vi "4-channel arduino.vi"() -> ()   [LabVIEW 2014]
uses:
  <vilib>/MakerHub/LINX/Public/Peripherals/Analog/Analog Read 1 Chan.vi
  <vilib>/MakerHub/LINX/LMH-LINX.lvlib
panel:
  out "Numeric":dbl
  in  "AI Channel 4":u8
  in  "AI Channel 3":u8
  in  "AI Channel 2":u8
  in  "AI Channel 1":u8
  in  "AI Channel 0":u8
  in  "Stop Button":bool
  out "Analog Data 0":dbl(graph)
  out "Loop Rate (Hz)":u32
  out "Analog Data 1":dbl(graph)
  out "Analog Data 2":dbl(graph)
  out "Analog Data 3":dbl(graph)
  out "Analog Data 4":dbl(graph)
  in  "Serial Port":refnum<visa-resource-name>
  # "Analog Data 0"
  # "Analog Data 1"
  # "Analog Data 4"
  # "Analog Data 2"
  # "Analog Data 3"
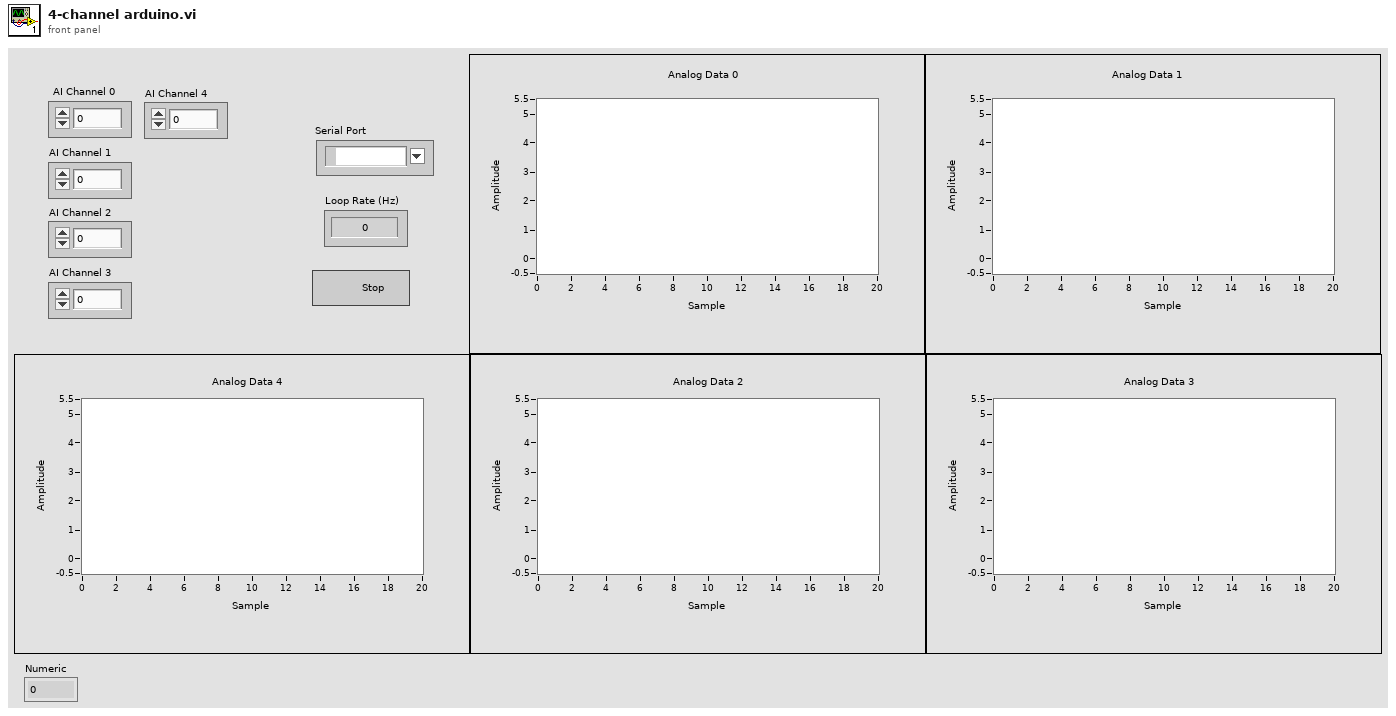
[diagram p1: front panel]
types:
  T1 = typedef "LMH-LINX.lvlib/LINX Ref.ctl" = cluster{"Platform":T2, "Interface":T3, "LINX Device Config":T4}
  T2 = typedef "LMH-LINX.lvlib/Platform.ctl" = enum16{"LINX", "myRIO"}
  T3 = typedef "LMH-LINX.lvlib/Interface.ctl" = enum16{"Serial", "TCP"}
  T4 = typedef "LMH-LINX.lvlib/Device.lvlib/LINX Device Config.ctl" = cluster{"Interface":T3, "COM Port":refnum<visa-resource-name>, "TCP Configuration":T5, "Device Family":u8, "Device ID":u8, "Device Name":string, "TCP Ref":refnum<k5>, "Channels":T6}
  T5 = typedef "LMH-LINX.lvlib/Device.lvlib/TCP Config.ctl" = cluster{"IP Address":string, "Port":u16}
  T6 = typedef "LMH-LINX.lvlib/Channels.ctl" = cluster{"DI":u8[], "DO":u8[], "AI":u8[], "AO":u8[], "PWM":u8[], "QE":u8[], "UART":u8[], "I2C 2":u8[], "SPI":u8[], "CAN":u8[], "Servo":u8[], "AI Ref (V)":dbl, "AO Ref (V)":dbl, "AO Resolution (Bits)":u8}
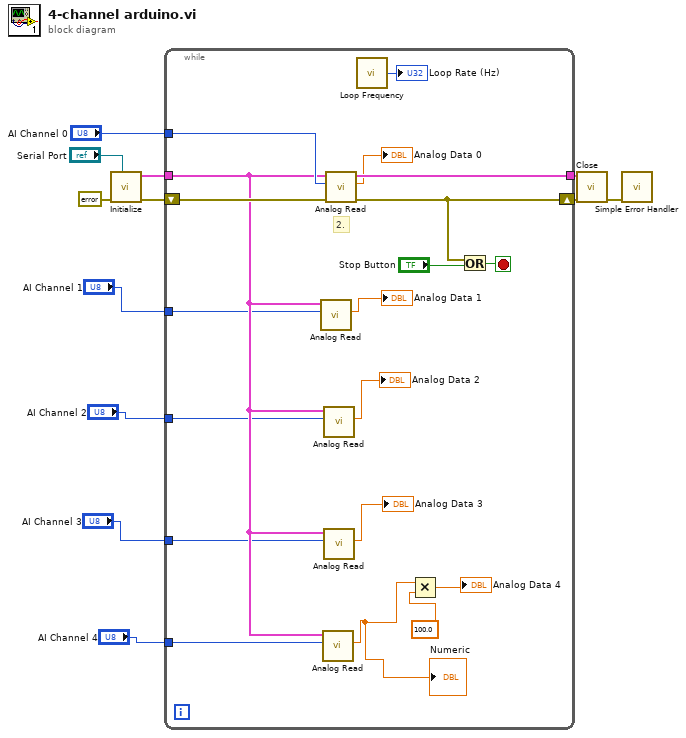
[diagram p0: block diagram]
diagram:
  n1 = call <vilib>:"Initialize.vi"("Serial Port"="Serial Port", "Error In"=errorcluster {"status"=FALSE, "code"=0, "source"=""}) -> ("Error Out"=w11:errorcluster, "LINX Ref"=w12:T1)  [unwired: 7 in, 1 out]
  n2 = while {
    tunnel: w12 -> [w23]
    tunnel: [w30] -> w10
    shift-right: [w27] -> w9
    shift-left: w11 -> [w31]
    tunnel: "AI Channel 0" -> [w25]
    tunnel: "AI Channel 1" -> [w22]
    tunnel: "AI Channel 2" -> [w21]
    tunnel: "AI Channel 3" -> [w20]
    tunnel: "AI Channel 4" -> [w19]
    stop <- w29 stop-if-true
    # "2."
    n3 = call-poly <vilib>:"Analog Read.vi"("Analog Channel"=w22, "LINX Resource"=w23) -> ("AI Value"=→"Analog Data 1":dbl)  [unwired: 6 in, 3 out]
    n4 = call-poly <vilib>:"Analog Read.vi"("Analog Channel"=w19, "LINX Resource"=w23) -> ("AI Value"=w14:dbl)  [unwired: 6 in, 3 out]
    "Numeric" <- w14
    n5 = call-poly <vilib>:"Analog Read.vi"("Analog Channel"=w21, "LINX Resource"=w23) -> ("AI Value"=→"Analog Data 2":dbl)  [unwired: 6 in, 3 out]
    n6 = call-poly <vilib>:"Analog Read.vi"("Analog Channel"=w20, "LINX Resource"=w23) -> ("AI Value"=→"Analog Data 3":dbl)  [unwired: 6 in, 3 out]
    n7 = call-poly <vilib>:"Analog Read.vi"("Error In"=w31, "Analog Channel"=w25, "LINX Resource"=w23) -> ("Error Out"=w27:errorcluster, "AI Value"=→"Analog Data 0":dbl, "LINX Resource"=w30:T1)  [unwired: 5 in, 1 out]
    n8 = call <vilib>:"Loop Frequency.vi"() -> ("Loop Rate (Hz)"=→"Loop Rate (Hz)":u32)
    n9 = Multiply(x=w14, y=100.0) -> (x*y=→"Analog Data 4":dbl)
    n10 = Or(x=w27, y="Stop Button") -> (x .or. y?=w29:bool)
  }
  n11 = call <vilib>:"Close.vi"("Error In"=w9, "LINX Resource"=w10) -> ("Error Out"=w7:errorcluster)  [unwired: 8 in, 1 out]
  n12 = call <vilib>:"Simple Error Handler.vi"("error in (no error)"=w7) -> ()  [unwired: 4 in, 5 out]
